vi "Set Magnet Vector Field.vi"(8 "error in (no error)":errorcluster, 9 "Target Rate (T/min)":dbl, 10 "Target Field (T)":dbl[](array[numeric]), 11 "Instrument.VRM in":refnum<class "Instrument.OxfordVRM.lvclass">) -> (0 "error out":errorcluster, 3 "Instrument.VRM out":refnum<class "Instrument.OxfordVRM.lvclass">)   [LabVIEW 2016, in "Instrument.OxfordVRM.lvclass"]
uses:
  Instrument.OxfordVRM.lvclass
  Typedefs/Instrument.Oxford1820.Commands-enum.ctl
  Typedefs/Instrument.Oxford1820.setMagnet-cluster.ctl
  Typedefs/VRM Targets--Cluster.ctl
  <userlib>/LevyLab/Levylab Instruments/Instrument Types/Cryostat/Typedefs/VRM Magnet Axis--Enum.ctl
  Typedefs/VRM Action-Axis--Cluster.ctl
  <instrlib>/Mercury iXX/Public/Libraries/Magnet/Controls/PSU Actions.ctl
  <instrlib>/Mercury iXX/Public/Libraries/Magnet.lvlib
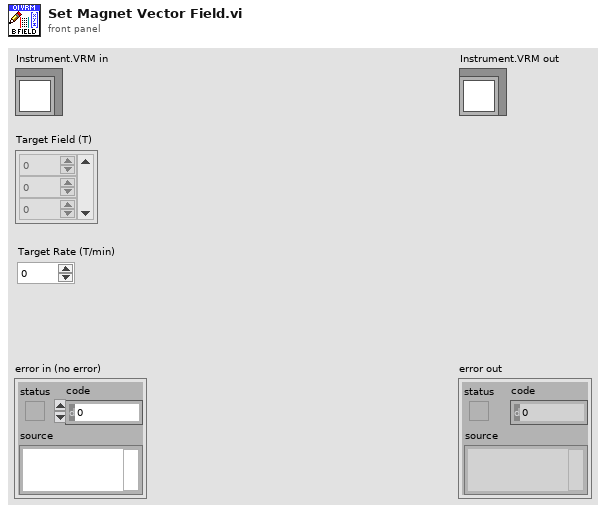
[diagram p1: front panel]
types:
  T1 = typedef "Instrument.OxfordVRM.lvclass/VRM Magnet Axis--Enum.ctl" = enum16{"Z", "X", "Y", "ALL"}
  T2 = typedef "Mercury iXX.lvlib/Magnet.lvlib/PSU Actions.ctl" = string
  T3 = typedef "Instrument.OxfordVRM.lvclass/VRM Action-Axis--Cluster.ctl" = cluster{"PSU Act Stat":T2, "Axis":T1}
  T4 = typedef "Instrument.OxfordVRM.lvclass/Instrument.Oxford1820.setMagnet-cluster.ctl" = cluster{"Target":T5}
  T5 = typedef "Instrument.OxfordVRM.lvclass/VRM Targets--Cluster.ctl" = cluster{"Field (T)":dbl, "Field Rate (T/min)":dbl, "Axis":T1}
  T6 = typedef "Instrument.OxfordVRM.lvclass/Instrument.Oxford1820.Commands-enum.ctl" = enum16{"setAction", "setTarget", "setMagnetField", "getStatus", "getTarget", "getMagnetField"}
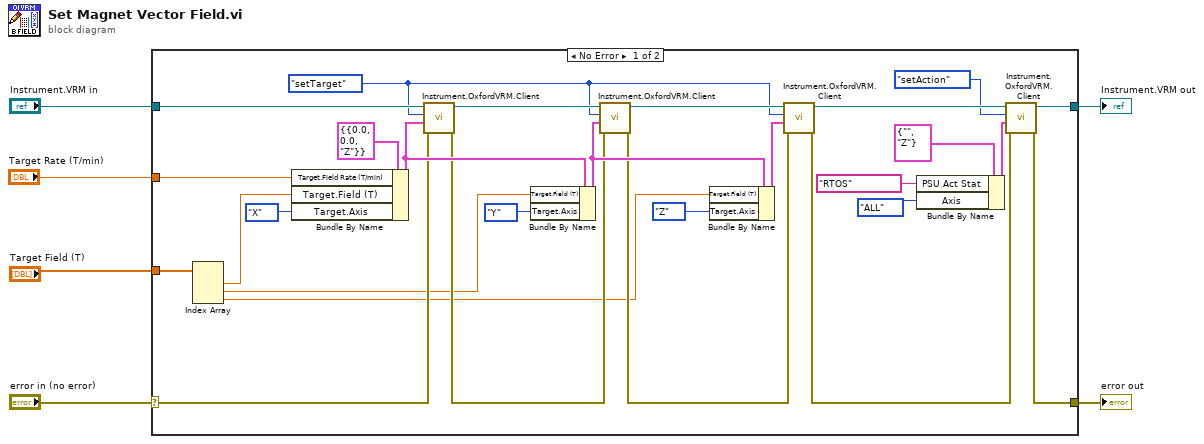
[diagram p0: block diagram]
diagram:
  n1 = case shown="No Error" "error in (no error)" {
    selector: "error in (no error)" -> [w22 w36]
    tunnel: [w14 w36] -> w6
    tunnel: "Instrument.VRM in" -> [w33 w35]
    tunnel: [w34 w35] -> w4
    tunnel: "Target Field (T)" -> [w32 _]
    tunnel: "Target Rate (T/min)" -> [w25 _]
    frame No Error {
      w17 = Instrument.Oxford1820.Commands-enum."setTarget" ("Commands")
      n2 = Index Array(array=w32) -> (element #1=w16:dbl, element #2=w19:dbl, element #3=w18:dbl)  [unwired: 3 in]
      n3 = Bundle By Name(cluster=T4 {"Target"={"Field (T)"=0.0, "Field Rate (T/min)"=0.0, "Axis"=enum."Z"}} ("output cluster"), "Target.Field Rate (T/min)"=w25, "Target.Field (T)"=w16, "Target.Axis"=VRM_Magnet_Axis--Enum."X" ("Axis")) -> (w26:T4)
      n4 = call "Instrument.OxfordVRM.Client.vi"("error in (no error)"=w22, "Data"=w26, "Commands"=w17, "Instrument.VRM in"=w33) -> ("error out"=w21:errorcluster, "Instrument.VRM out"=w30:refnum<class "Instrument.OxfordVRM.lvclass">)  [unwired: 5 in, 1 out]
      n5 = Bundle By Name(cluster=w26, "Target.Field (T)"=w19, "Target.Axis"=VRM_Magnet_Axis--Enum."Y" ("Axis")) -> (w23:T4)
      n6 = call "Instrument.OxfordVRM.Client.vi"("error in (no error)"=w21, "Data"=w23, "Commands"=w17, "Instrument.VRM in"=w30) -> ("error out"=w20:errorcluster, "Instrument.VRM out"=w31:refnum<class "Instrument.OxfordVRM.lvclass">)  [unwired: 5 in, 1 out]
      n7 = Bundle By Name(cluster=w23, "Target.Field (T)"=w18, "Target.Axis"=VRM_Magnet_Axis--Enum."Z" ("Axis")) -> (w24:T4)
      n8 = call "Instrument.OxfordVRM.Client.vi"("error in (no error)"=w20, "Data"=w24, "Commands"=w17, "Instrument.VRM in"=w31) -> ("error out"=w15:errorcluster, "Instrument.VRM out"=w29:refnum<class "Instrument.OxfordVRM.lvclass">)  [unwired: 5 in, 1 out]
      n9 = Bundle By Name(cluster=T3 {"PSU Act Stat"="", "Axis"=enum."Z"} ("Action"), "PSU Act Stat"=T2 "RTOS", "Axis"=VRM_Magnet_Axis--Enum."ALL") -> (w7:T3)
      n10 = call "Instrument.OxfordVRM.Client.vi"("error in (no error)"=w15, "Data"=w7, "Commands"=Instrument.Oxford1820.Commands-enum."setAction", "Instrument.VRM in"=w29) -> ("error out"=w14:errorcluster, "Instrument.VRM out"=w34:refnum<class "Instrument.OxfordVRM.lvclass">)  [unwired: 5 in, 1 out]
    }
    frame Error {
    }
  }
  "Instrument.VRM out" <- w4
  "error out" <- w6
